vi "Get Detector Trace Auto Enabled.vi"(8 "error in (no error)":errorcluster {"code" format="%.0x"}, 9 "TraceNo":i32=1 caption="TraceNo (1)" format="%.0g", 11 "instrument handle":refnum<k15>) -> (0 "error out":errorcluster {"code" format="%.0x"}, 2 "RetVal":bool, 3 "instrument handle out":refnum<k15>)   [LabVIEW 2009, in "Keysight XSAn.lvlib"]
doc: "Queries if the detector selection mode for the currently selected trace is set to Auto.\n\nSupported Models: All supported"
uses:
  <instrlib>/Keysight XSAn/Keysight XSAn.lvlib
  AgXSAn.dll
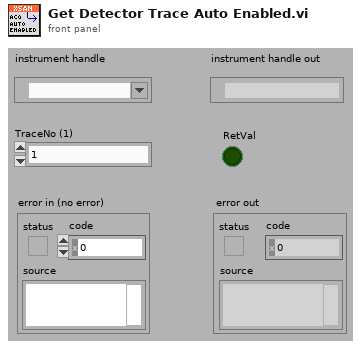
[diagram p1: front panel]
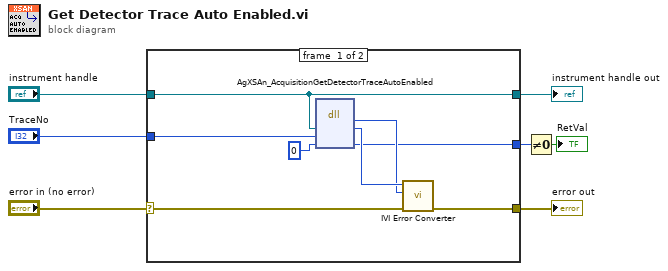
[diagram p0: block diagram]
diagram:
  n1 = case shown="No Error" "error in (no error)" {
    selector: "error in (no error)" -> [w13 w17]
    tunnel: [w12 w17] -> w7
    tunnel: "instrument handle" -> [w8 w16]
    tunnel: "TraceNo" -> [w11 _]
    tunnel: [w9 _] -> w3
    tunnel: [w8 w16] -> w1
    frame #0 {
      n2 = dll-call lib="AgXSAn**.dll" fn="AgXSAn_AcquisitionGetDetectorTraceAutoEnabled"("Vi"=w8, "TraceNo"=w11, "RetVal"=i16 0) -> (w14:i32, "Vi"=w15:u32, "RetVal"=w9:i16)  [unwired: 4 in, 2 out]
      n3 = call <instrlib>:"IVI Error Converter.vi"("error in (no error)"=w13, "IVI error code (0)"=w14, "instrument handle"=w15) -> ("error out"=w12:errorcluster)  [unwired: 7 in, 1 out]
    }
    frame #1 {
    }
  }
  "error out" <- w7
  "instrument handle out" <- w1
  n4 = Not Equal To 0?(x=w3) -> (x != 0?=→"RetVal":bool)
